vi "SMSMagnet.set modified data.vi"(0 "i ref in":refnum<vi>, 2 "i attribute":T1, 5 "error in (no error)":errorcluster) -> (14 "i ref out":refnum<vi>, 19 "error out":errorcluster)   [LabVIEW 2014, in "SMSMagnet.lvlib"]
doc: "Writes the data into the attribute of an object. Then, the attribute dara are unlocked using the \"release\" method. Prior to calling THIS method, the attribute data must have been locked using the methods \"lock\" or \"get data to modify\".\n\n\nLicense Agreement for this software:\n\nCopyright (C)\nGesellschaft für Schwerionenforschung, GSI\nPlanckstr. 1\n64291 Darmstadt\nGermany\n\nContact: D.Beck@gsi.de \n\nThis program is free software; you can redistribute it and/or modify it under the terms of the GNU General Public License as published by the Free Software Foundation; either version 2 of the license, or (at your option) any later version.\n\nThis program is distributed in the hope that it will be useful, but WITHOUT ANY WARRANTY; without even the implied warranty of MERCHANTABILITY or FITNESS FOR A PARTICULAR PURPOSE. See the GNU General License for more details (http://www.gnu.org).\n\nGesellschaft für Schwerionenforschung, GSI\nPlanckstr. 1, 64291 Darmstadt, Germany\nFor all questions and ideas contact: M.Richter@gsi.de, H.Brand@gsi.de or D.Beck@gsi.de.\nLast update: 17-JUN-2004"
uses:
  SMSMagnet.lvlib
  SMSMagnet.i attribute.ctl
  CS_Core/CSObj/CSObj.lvlib
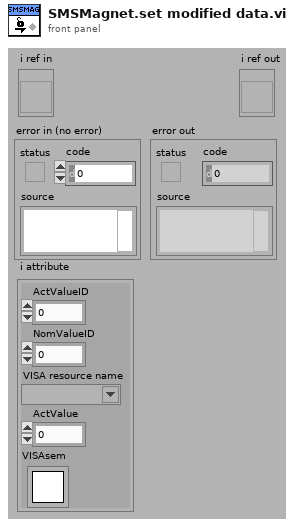
[diagram p1: front panel]
types:
  T1 = typedef "SMSMagnet.lvlib/SMSMagnet.i attribute.ctl" = cluster{"ActValueID":i32, "NomValueID":i32, "VISA resource name":refnum<visa-resource-name>, "ActValue":dbl, "VISAsem":T2}
  T2 = typedef "Semaphore RefNum" = refnum<k1>
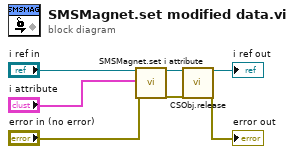
[diagram p0: block diagram]
diagram:
  n1 = call "SMSMagnet.set i attribute.vi"("i ref in"="i ref in", "i attribute"="i attribute", "error in (no error)"="error in (no error)") -> ("i ref out"=w4:refnum<vi>, "error out"=w3:errorcluster)  [unwired: 15 in]
  n2 = call "CSObj.release.vi"("i ref in"=w4, "error in (no error)"=w3) -> ("i ref out"=→"i ref out":refnum<vi>, "error out"=→"error out":errorcluster)  [unwired: 16 in]
